vi "Excel_Font_Wizard.vi"(3 "error in (no error)":errorcluster, 4 "font in":T1={"font name"="", "font size"=0.0, "bold"=0, "italic"=0, "underline"=0, "strike through"=0, "font color"=16777216} caption="font" {"font size" format="%0.2f"; "strike through" items=["Unchanged", "Yes", "No"]; "underline" items=["Unchanged", "Yes", "No"]; "italic" items=["Unchanged", "Yes", "No"]; "bold" items=["Unchanged", "Yes", "No"]}, 5 "Minimize Excel":bool) -> (0 "error out":errorcluster, 1 "font out":T1={"font name"="", "font size"=0.0, "bold"=0, "italic"=0, "underline"=0, "strike through"=0, "font color"=16777216} caption="font" {"font size" format="%0.2f"; "strike through" items=["Unchanged", "Yes", "No"]; "underline" items=["Unchanged", "Yes", "No"]; "italic" items=["Unchanged", "Yes", "No"]; "bold" items=["Unchanged", "Yes", "No"]})   [LabVIEW 2020, in "NI_ReportGenerationToolkit.lvlib"]
uses:
  <vilib>/addons/_office/NI_ReportGenerationToolkit.lvlib
  <vilib>/addons/_office/_exclsub.llb/font.ctl
  <vilib>/Utility/NIReport.llb/Excel/NI_Excel.lvclass
  <vilib>/Utility/NIReport.llb/NI_report.lvclass
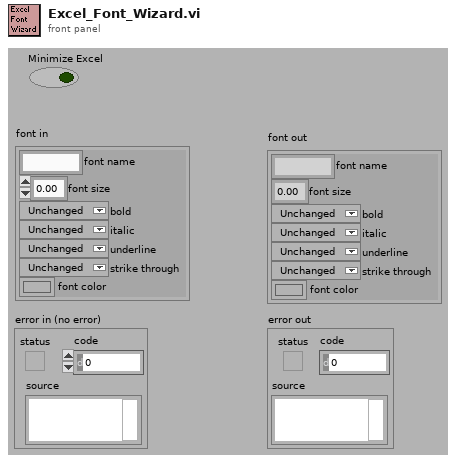
[diagram p1: front panel]
types:
  T1 = typedef "NI_ReportGenerationToolkit.lvlib/font.ctl" = cluster{"font name":string, "font size":dbl, "bold":u16, "italic":u16, "underline":u16, "strike through":u16, "font color":u32}
  T2 = enum16{"Standard Report", "HTML", "Word", "Excel"}
  T3 = cluster{"Excel._Application":refnum<k7>, "Excel._Workbook":refnum<k7>, "Excel._Worksheet":refnum<k7>, "Excel.Sheets":refnum<k7>, "Excel.Shapes":refnum<k7>}
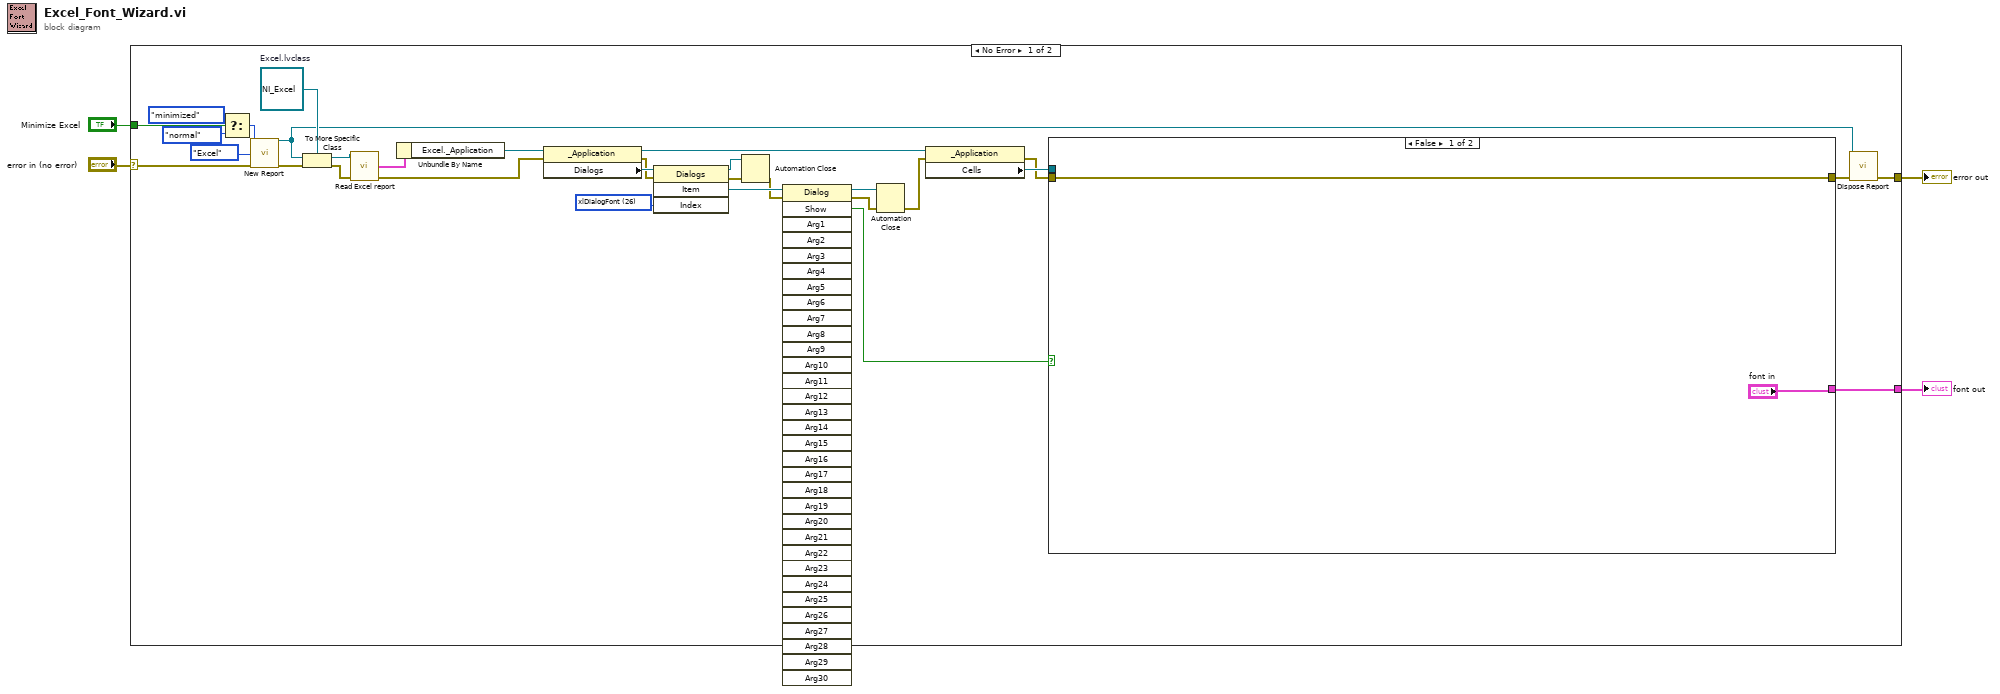
[diagram p0: block diagram]
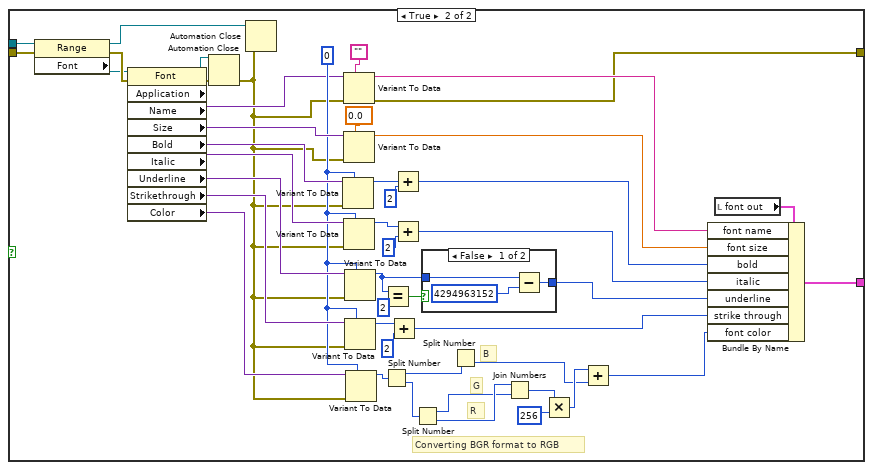
[diagram p2: hidden frame]
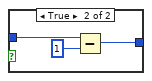
[diagram p3: hidden frame]
diagram:
  n1 = case shown="No Error" "error in (no error)" {
    selector: "error in (no error)" -> [w14 w90]
    tunnel: [w30 _] -> w4
    tunnel: [w12 w90] -> w3
    tunnel: "Minimize Excel" -> [w20 _]
    frame No Error {
      w10 = refnum<class "NI_Excel.lvclass"> refnum  # Excel.lvclass
      w35 = 26 items=["xlDialogOpen"=1, "xlDialogOpenLinks"=2, "xlDialogSaveAs"=5, "xlDialogFileDelete"=6, "xlDialogPageSetup"=7, "xlDialogPrint"=8, "xlDialogPrinterSetup"=9, "xlDialogArrangeAll"=12, "xlDialogWindowSize"=13, "xlDialogWindowMove"=14, "xlDialogRun"=17, "xlDialogSetPrintTitles"=23, "xlDialogFont"=26, "xlDialogDisplay"=27, "xlDialogProtectDocument"=28, "xlDialogCalculation"=32, "xlDialogExtract"=35, "xlDialogDataDelete"=36, "xlDialogSort"=39, "xlDialogDataSeries"=40, "xlDialogTable"=41, "xlDialogFormatNumber"=42, "xlDialogAlignment"=43, "xlDialogStyle"=44, "xlDialogBorder"=45, "xlDialogCellProtection"=46, "xlDialogColumnWidth"=47, "xlDialogClear"=52, "xlDialogPasteSpecial"=53, "xlDialogEditDelete"=54, "xlDialogInsert"=55, "xlDialogPasteNames"=58, "xlDialogDefineName"=61, "xlDialogCreateNames"=62, "xlDialogFormulaGoto"=63, "xlDialogFormulaFind"=64, "xlDialogGalleryArea"=67, "xlDialogGalleryBar"=68, "xlDialogGalleryColumn"=69, "xlDialogGalleryLine"=70, "xlDialogGalleryPie"=71, "xlDialogGalleryScatter"=72, "xlDialogCombination"=73, "xlDialogGridlines"=76, "xlDialogAxes"=78, "xlDialogAttachText"=80, "xlDialogPatterns"=84, "xlDialogMainChart"=85, "xlDialogOverlay"=86, "xlDialogScale"=87, "xlDialogFormatLegend"=88, "xlDialogFormatText"=89, "xlDialogParse"=91, "xlDialogUnhide"=94, "xlDialogWorkspace"=95, "xlDialogActivate"=103, "xlDialogCopyPicture"=108, "xlDialogDeleteName"=110, "xlDialogDeleteFormat"=111, "xlDialogNew"=119, "xlDialogRowHeight"=127, "xlDialogFormatMove"=128, "xlDialogFormatSize"=129, "xlDialogFormulaReplace"=130, "xlDialogSelectSpecial"=132, "xlDialogApplyNames"=133, "xlDialogReplaceFont"=134, "xlDialogSplit"=137, "xlDialogOutline"=142, "xlDialogSaveWorkbook"=145, "xlDialogCopyChart"=147, "xlDialogFormatFont"=150, "xlDialogNote"=154, "xlDialogSetUpdateStatus"=159, "xlDialogColorPalette"=161, "xlDialogChangeLink"=166, "xlDialogAppMove"=170, "xlDialogAppSize"=171, "xlDialogMainChartType"=185, "xlDialogOverlayChartType"=186, "xlDialogOpenMail"=188, "xlDialogSendMail"=189, "xlDialogStandardFont"=190, "xlDialogConsolidate"=191, "xlDialogSortSpecial"=192, "xlDialogGallery3dArea"=193, "xlDialogGallery3dColumn"=194, "xlDialogGallery3dLine"=195, "xlDialogGallery3dPie"=196, "xlDialogView3d"=197, "xlDialogGoalSeek"=198, "xlDialogWorkgroup"=199, "xlDialogFillGroup"=200, "xlDialogUpdateLink"=201, "xlDialogPromote"=202, "xlDialogDemote"=203, "xlDialogShowDetail"=204, "xlDialogObjectProperties"=207, "xlDialogSaveNewObject"=208, "xlDialogApplyStyle"=212, "xlDialogAssignToObject"=213, "xlDialogObjectProtection"=214, "xlDialogCreatePublisher"=217, "xlDialogSubscribeTo"=218, "xlDialogShowToolbar"=220, "xlDialogPrintPreview"=222, "xlDialogEditColor"=223, "xlDialogFormatMain"=225, "xlDialogFormatOverlay"=226, "xlDialogEditSeries"=228, "xlDialogDefineStyle"=229, "xlDialogGalleryRadar"=249, "xlDialogEditionOptions"=251, "xlDialogZoom"=256, "xlDialogInsertObject"=259, "xlDialogSize"=261, "xlDialogMove"=262, "xlDialogFormatAuto"=269, "xlDialogGallery3dBar"=272, "xlDialogGallery3dSurface"=273, "xlDialogCustomizeToolbar"=276, "xlDialogWorkbookAdd"=281, "xlDialogWorkbookMove"=282, "xlDialogWorkbookCopy"=283, "xlDialogWorkbookOptions"=284, "xlDialogSaveWorkspace"=285, "xlDialogChartWizard"=288, "xlDialogAssignToTool"=293, "xlDialogPlacement"=300, "xlDialogFillWorkgroup"=301, "xlDialogWorkbookNew"=302, "xlDialogScenarioCells"=305, "xlDialogScenarioAdd"=307, "xlDialogScenarioEdit"=308, "xlDialogScenarioSummary"=311, "xlDialogPivotTableWizard"=312, "xlDialogPivotFieldProperties"=313, "xlDialogOptionsCalculation"=318, "xlDialogOptionsEdit"=319, "xlDialogOptionsView"=320, "xlDialogAddinManager"=321, "xlDialogMenuEditor"=322, "xlDialogAttachToolbars"=323, "xlDialogOptionsChart"=325, "xlDialogVbaInsertFile"=328, "xlDialogVbaProcedureDefinition"=330, "xlDialogRoutingSlip"=336, "xlDialogMailLogon"=339, "xlDialogInsertPicture"=342, "xlDialogGalleryDoughnut"=344, "xlDialogChartTrend"=350, "xlDialogWorkbookInsert"=354, "xlDialogOptionsTransition"=355, "xlDialogOptionsGeneral"=356, "xlDialogFilterAdvanced"=370, "xlDialogMailNextLetter"=378, "xlDialogDataLabel"=379, "xlDialogInsertTitle"=380, "xlDialogFontProperties"=381, "xlDialogMacroOptions"=382, "xlDialogWorkbookUnhide"=384, "xlDialogWorkbookName"=386, "xlDialogGalleryCustom"=388, "xlDialogAddChartAutoformat"=390, "xlDialogChartAddData"=392, "xlDialogTabOrder"=394, "xlDialogSubtotalCreate"=398, "xlDialogWorkbookTabSplit"=415, "xlDialogWorkbookProtect"=417, "xlDialogScrollbarProperties"=420, "xlDialogPivotShowPages"=421, "xlDialogTextToColumns"=422, "xlDialogFormatCharttype"=423, "xlDialogPivotFieldGroup"=433, "xlDialogPivotFieldUngroup"=434, "xlDialogCheckboxProperties"=435, "xlDialogLabelProperties"=436, "xlDialogListboxProperties"=437, "xlDialogEditboxProperties"=438, "xlDialogOpenText"=441, "xlDialogPushbuttonProperties"=445, "xlDialogFilter"=447, "xlDialogFunctionWizard"=450, "xlDialogSaveCopyAs"=456, "xlDialogOptionsListsAdd"=458, "xlDialogSeriesAxes"=460, "xlDialogSeriesX"=461, "xlDialogSeriesY"=462, "xlDialogErrorbarX"=463, "xlDialogErrorbarY"=464, "xlDialogFormatChart"=465, "xlDialogSeriesOrder"=466, "xlDialogMailEditMailer"=470, "xlDialogStandardWidth"=472, "xlDialogScenarioMerge"=473, "xlDialogProperties, xlDialogSummaryInfo"=474, "xlDialogFindFile"=475, "xlDialogActiveCellFont"=476, "xlDialogVbaMakeAddin"=478, "xlDialogFileSharing"=481, "xlDialogAutoCorrect"=485, "xlDialogCustomViews"=493, "xlDialogInsertNameLabel"=496, "xlDialogSeriesShape"=504, "xlDialogChartOptionsDataLabels"=505, "xlDialogChartOptionsDataTable"=506, "xlDialogSetBackgroundPicture"=509, "xlDialogDataValidation"=525, "xlDialogChartType"=526, "xlDialogChartLocation"=527, "_xlDialogPhonetic"=538, "xlDialogChartSourceData"=540, "_xlDialogChartSourceData"=541, "xlDialogSeriesOptions"=557, "xlDialogPivotTableOptions"=567, "xlDialogPivotSolveOrder"=568, "xlDialogPivotCalculatedField"=570, "xlDialogPivotCalculatedItem"=572, "xlDialogConditionalFormatting"=583, "xlDialogInsertHyperlink"=596, "xlDialogProtectSharing"=620, "xlDialogOptionsME"=647, "xlDialogPublishAsWebPage"=653, "xlDialogPhonetic"=656, "xlDialogNewWebQuery"=667, "xlDialogImportTextFile"=666, "xlDialogExternalDataProperties"=530, "xlDialogWebOptionsGeneral"=683, "xlDialogWebOptionsFiles"=684, "xlDialogWebOptionsPictures"=685, "xlDialogWebOptionsEncoding"=686, "xlDialogWebOptionsFonts"=687, "xlDialogPivotClientServerSet"=689, "xlDialogPropertyFields"=754, "xlDialogSearch"=731, "xlDialogEvaluateFormula"=709, "xlDialogDataLabelMultiple"=723, "xlDialogChartOptionsDataLabelMultiple"=724, "xlDialogErrorChecking"=732, "xlDialogWebOptionsBrowsers"=773] ("Index")
      n2 = Select(t=enum16{"maximized", "minimized", "normal"}."minimized" ("window state (normal)"), s=w20, f=enum16{"maximized", "minimized", "normal"}."normal" ("window state (normal)")) -> (s? t:f=w15:enum16{"maximized", "minimized", "normal"})
      n3 = call <vilib>:"New Report.vi"("window state (normal)"=w15, "report type"=T2."Excel" ("report type (standard)"), "error in (no error)"=w14) -> ("report out"=w5:refnum<class "NI_report.lvclass">, "error out"=w7:errorcluster)  [unwired: 3 in, 8 out]
      n4 = To More Specific Class(target class=w10, reference=w5, error in=w7) -> (specific class reference=w11:refnum<class "NI_Excel.lvclass">, error out=w8:errorcluster)
      n5 = call-dynamic "Read Excel report.vi"("report in"=w11, "error in (no error)"=w8) -> ("Excel report"=w9:T3, "error out"=w6:errorcluster)  [unwired: 11 in, 1 out]
      n6 = Unbundle By Name(w9) -> ("Excel._Application"=w17:refnum<k7>)
      n7 = property class="_Application"(reference=w17, error in=w6) -> (reference out=w22:refnum<k7>, error out=w26:errorcluster, "Dialogs"=w27:refnum<k7>)
      n8 = invoke class="Dialogs" method="Item"(reference=w27, error in=w26, "Index"=w35) -> (reference out=w24:refnum<k7>, error out=w23:errorcluster, "Item"=w34:refnum<k7>)  [unwired: 1 in, 1 out]
      n9 = Automation Close(3:w23, 5:w24) -> (0:w25:errorcluster)
      n10 = invoke class="Dialog" method="Show"(reference=w34, error in=w25) -> (reference out=w29:refnum<k7>, error out=w28:errorcluster, "Show"=w31:bool)  [unwired: 31 in, 30 out]
      n11 = Automation Close(3:w28, 5:w29) -> (0:w21:errorcluster)
      n12 = property class="_Application"(reference=w22, error in=w21) -> (error out=w32:errorcluster, "Cells"=w33:refnum<k7>)  [unwired: 1 out]
      n13 = case shown="False" w31 {
        tunnel: w33 -> [_ w83]
        tunnel: w32 -> [w36 w41]
        tunnel: ["font in" w46] -> w30
        tunnel: [w36 w42] -> w13
        frame False {
        }
        frame True {
          w73 = u32 0
          # "Converting BGR format to RGB"
          # "R"
          # "G"
          # "B"
          n14 = property class="Range"(reference=w83, error in=w41) -> (reference out=w43:refnum<k7>, error out=w82:errorcluster, "Font"=w81:refnum<k7>)
          n15 = property class="Font" props=["Application", "Name", "Size", "Bold", "Italic", "Underline", "Strikethrough", "Color"](reference=w81, error in=w82) -> (reference out=w44:refnum<k7>, error out=w45:errorcluster, "Name"=w39:variant, "Size"=w80:variant, "Bold"=w79:variant, "Italic"=w78:variant, "Underline"=w77:variant, "Strikethrough"=w76:variant, "Color"=w75:variant)  [unwired: 1 out]
          n16 = Automation Close(3:w45, 5:w44) -> (0:w38:errorcluster)
          n17 = Automation Close(3:w38, 5:w43) -> ()  [unwired: 1 out]
          n18 = Variant To Data(error in=w38, type=w73, Variant=w79) -> (data=w70:u32)  [unwired: 1 out]
          n19 = Variant To Data(error in=w38, type="", Variant=w39) -> (data=w72:string, error out=w42:errorcluster)
          n20 = Variant To Data(error in=w38, type=0.0, Variant=w80) -> (data=w71:dbl)  [unwired: 1 out]
          n21 = Variant To Data(error in=w38, type=w73, Variant=w78) -> (data=w65:u32)  [unwired: 1 out]
          n22 = Variant To Data(error in=w38, type=w73, Variant=w77) -> (data=w48:u32)  [unwired: 1 out]
          n23 = Variant To Data(error in=w38, type=w73, Variant=w76) -> (data=w62:u32)  [unwired: 1 out]
          n24 = Variant To Data(error in=w38, type=w73, Variant=w75) -> (data=w60:u32)  [unwired: 1 out]
          n25 = Split Number(x=w60) -> (hi(x)=w58:u16, lo(x)=w59:u16)
          n26 = Equal?(x=w48, y=u32 2) -> (x = y?=w49:bool)
          n27 = Add(x=w62, y=2) -> (x+y=w63:u32)
          n28 = Add(x=w70, y=2) -> (x+y=w68:u32)
          n29 = Add(x=w65, y=2) -> (x+y=w66:u32)
          n30 = Split Number(x=w59) -> (hi(x)=w56:u8, lo(x)=w57:u8)
          n31 = case shown="False" w49 {
            tunnel: w48 -> [w85 w89]
            tunnel: [w86 w87] -> w50
            frame False {
              n32 = Subtract(x=w85, y=u32 4294963152) -> (x-y=w86:u32)
            }
            frame True {
              n33 = Subtract(x=w89, y=u32 1) -> (x-y=w87:u32)
            }
          }
          n34 = Split Number(x=w58) -> (lo(x)=w52:u8)  [unwired: 1 out]
          n35 = Join Numbers(hi=w57, lo=w56) -> ((hi.lo)=w55:u16)
          n36 = Multiply(x=w55, y=u32 256) -> (x*y=w53:u32)
          n37 = Add(x=w53, y=w52) -> (x+y=w51:u32)
          n38 = local read "font out"() -> (w69:T1)
          n39 = Bundle By Name(cluster=w69, "font name"=w72, "font size"=w71, "bold"=w68, "italic"=w66, "underline"=w50, "strike through"=w63, "font color"=w51) -> (w46:T1)
        }
      }
      n40 = call-dynamic "Dispose Report.vi"("report in"=w5, "error in (no error)"=w13) -> ("error out"=w12:errorcluster)  [unwired: 13 in]
    }
    frame Error {
    }
  }
  "error out" <- w3
  "font out" <- w4
